vi "MongoDB.RemoveUser.vi"(8 "error in (no error)":errorcluster, 10 "username":string, 11 "MongoDB.Database in":refnum<class "MongoDB.Database.lvclass">) -> (0 "error out":errorcluster, 3 "MongoDB.Database out":refnum<class "MongoDB.Database.lvclass">)   [LabVIEW 2014, in "MongoDB.Database.lvclass"]
uses:
  MongoDB.Database.lvclass
  MongoDB.Database.lvclass/MongoDB.Database.ctl
  C:/Users/Richard/Documents/GitHub/mongo-labview-driver/CSharp/bin/MongoDB.Driver.Legacy.dll
  CSharp/bin/MongoDB.Driver.Legacy.dll
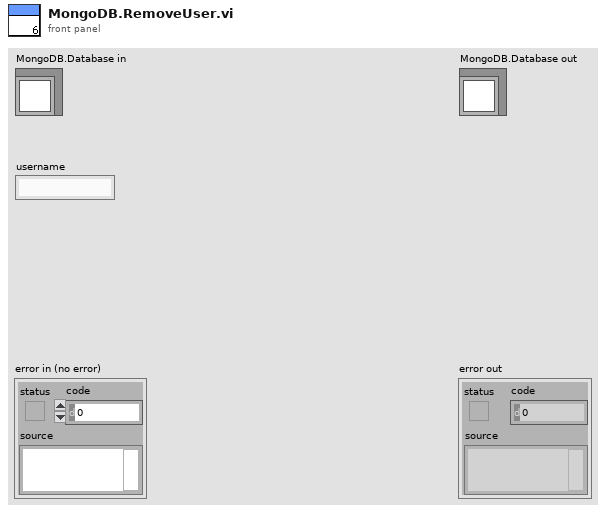
[diagram p1: front panel]
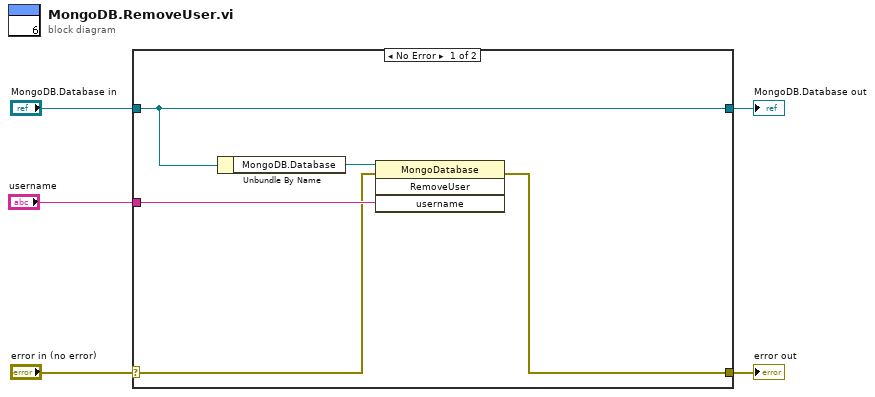
[diagram p0: block diagram]
diagram:
  n1 = case shown="No Error" "error in (no error)" {
    selector: "error in (no error)" -> [w7 w12]
    tunnel: [w6 w12] -> w4
    tunnel: [w10 w11] -> w2
    tunnel: "MongoDB.Database in" -> [w10 w11]
    tunnel: "username" -> [w8 _]
    frame No Error {
      n2 = Unbundle By Name(w10) -> ("MongoDB.Database"=w9:refnum<k24>)
      n3 = invoke class="MongoDatabase" method="RemoveUser"(reference=w9, error in=w7, "username"=w8) -> (error out=w6:errorcluster)  [unwired: 1 in, 3 out]
    }
    frame Error {
    }
  }
  "error out" <- w4
  "MongoDB.Database out" <- w2
